vi "Desktop Main.vi"() -> ()   [LabVIEW 2020]
doc: "This template is the Desktop portion of the touch panel template. It is based off of the Queued Message Handler design pattern.\n\nThe Event Handling Loop generates messages based on user interface actions.\n\nThe Message Handling Loop processes messages generated by the Event Handling Loop, or by other messages. The messages are string values, so new messages can be added easily to the Message Cases case structure in the Message Handling Loop. Each message cluster can also provide an optional value for Message Data, which is a variant that can be converted to whatever message-specific data is required.\n\nData is transfered to and from the touch panel target with the use of Shared Variables."
uses:
  controls/UI Data.ctl
  support/Message Queue/Enqueue Message (Single).vi
  <vilib>/Utility/error.llb/Error Cluster From Error Code.vi
  <vilib>/ErrorRing/Error Ring.xnode
  support/Message Queue/Message Queue.lvlib
  support/User Event - Stop/User Event - Stop.lvlib
panel:
  out "Data":dbl(graph)
  in  "Alarm Threshold <Replace Me>":dbl=5.0 format="%#_13g"
  in  "Exit":bool
  # "This template is based off of the Queued Message Handler design pattern.\n\nSee the Queued Message Handler documentation for more information on how to use this design pattern."
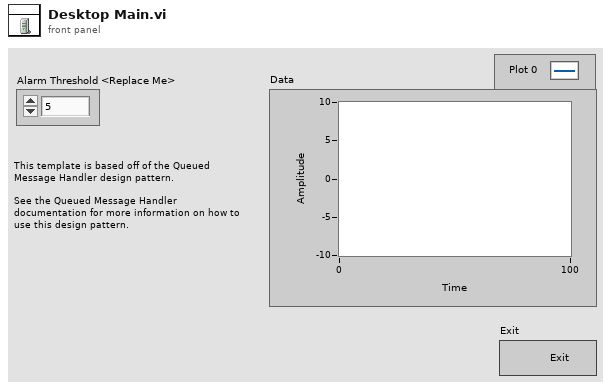
[diagram p1: front panel]
types:
  T1 = typedef "UI Data.ctl" = cluster{"Alarm Threshold <Replace Me>":refnum<vi>, "Exit Button Ref":refnum<vi>}
  T2 = typedef "Message Queue.lvlib/All Message Queues.ctl" = cluster{"UI":refnum<queue>}
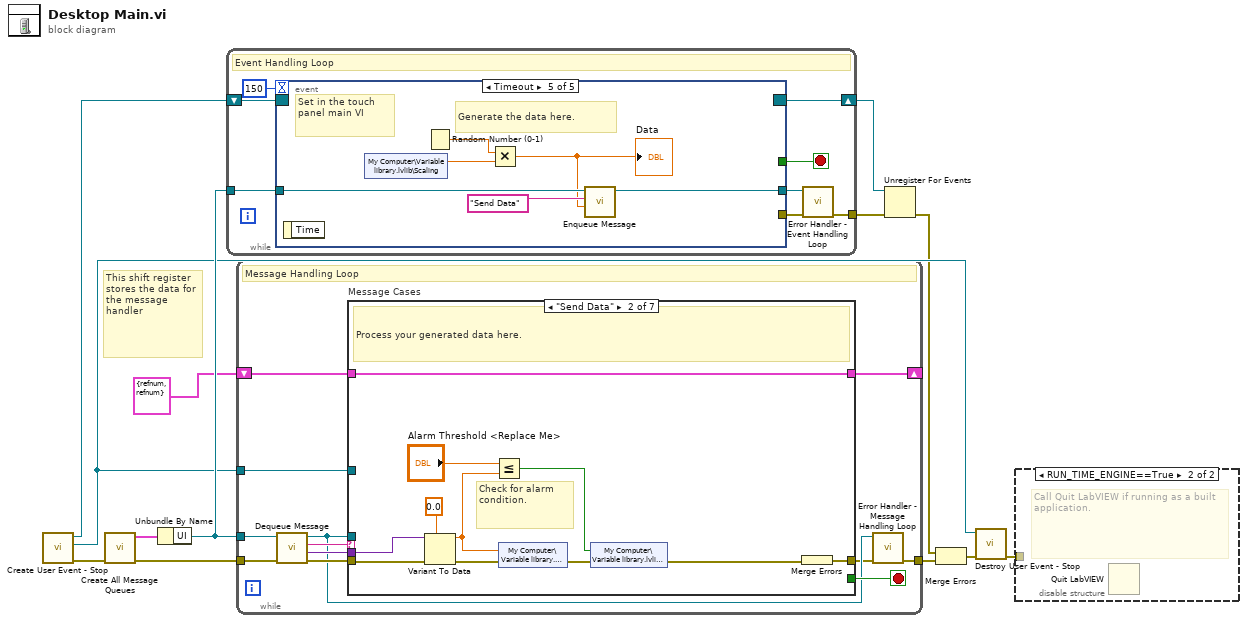
[diagram p0: block diagram]
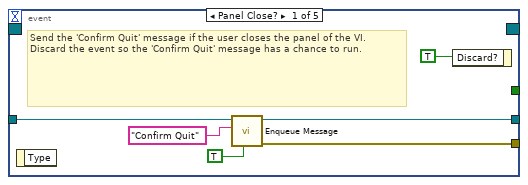
[diagram p3: hidden frame]
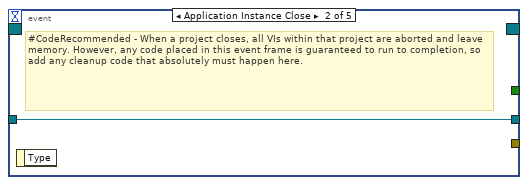
[diagram p4: hidden frame]
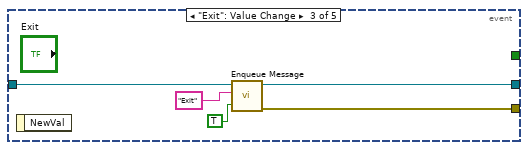
[diagram p5: hidden frame]
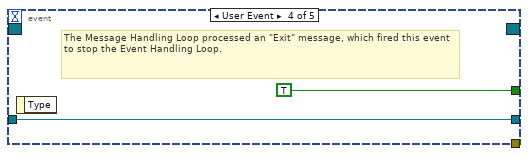
[diagram p6: hidden frame]
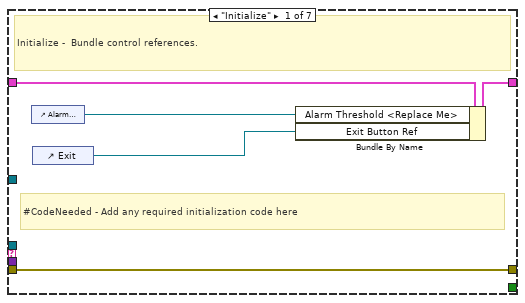
[diagram p7: hidden frame]
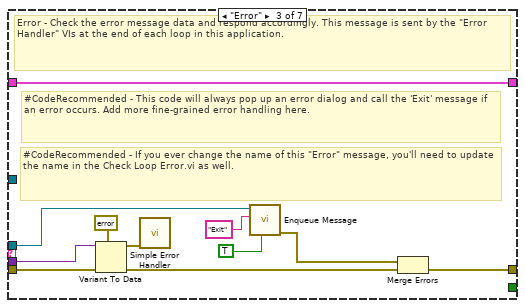
[diagram p8: hidden frame]
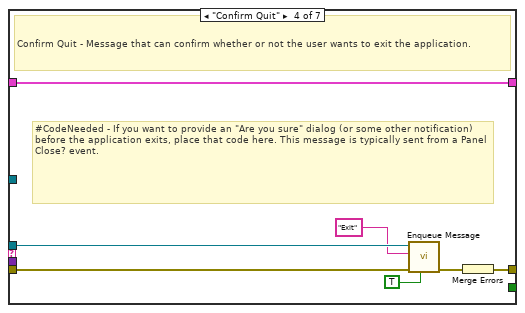
[diagram p9: hidden frame]
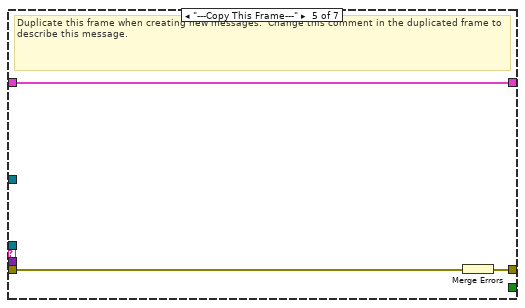
[diagram p10: hidden frame]
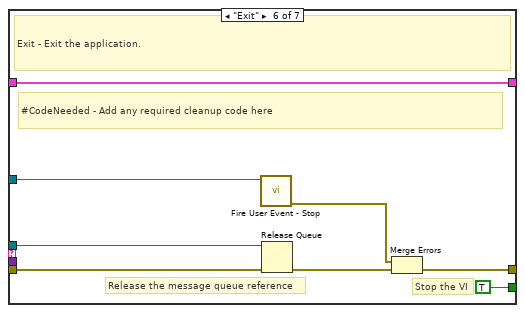
[diagram p11: hidden frame]
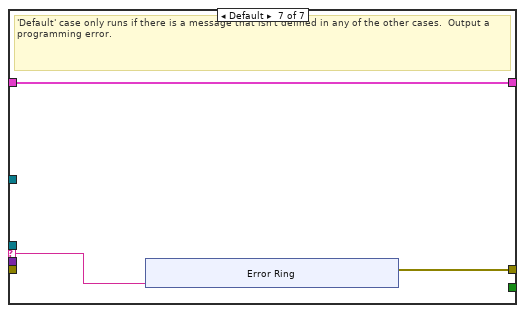
[diagram p12: hidden frame]
diagram:
  # "This shift register stores the data for the message handler"
  n1 = call "Create User Event - Stop.vi"() -> ("error out"=w8:errorcluster, "User Event - Stop"=w6:refnum<user-event>, "Stop Event Registration Refnum"=w9:refnum<event-registration>)  [unwired: 9 in]
  n2 = call "Create All Message Queues.vi"("error in (no error)"=w8) -> ("error out"=w13:errorcluster, "Message Queues out"=w12:T2)  [unwired: 9 in]
  n3 = Unbundle By Name(w12) -> ("UI"=w10:refnum<queue>)
  n4 = while {
    tunnel: w10 -> [w21]
    shift-right: [w19] -> w4
    shift-left: w9 -> [w20]
    tunnel: [w15] -> w1
    stop <- w17 stop-if-true
    # "Event Handling Loop"
    n5 = event shown="[4] Timeout" {
      selector: w20 -> [_ _ _ _ _]
      dyn-events: [_ _ _ _ _] -> w19
      timeout: 150 -> [_ _ _ _ _]
      tunnel: [_ _ _ TRUE ("Discard?") _] -> w17
      tunnel: w21 -> [w26 w28 w33 w35 w41]
      tunnel: [w25 _ w32 _ _] -> w18
      tunnel: [w24 w28 w31 w35 w40] -> w16
      event Panel Close? {
        # "Send the 'Confirm Quit' message if the user closes the panel of the VI. Discard the event so the 'Confirm Quit' message has a chance to run."
        n6 = event-data() -> ()  [unwired: 1 in, 1 out]
        n7 = call-poly "Enqueue Message.vi"("Priority Message? (F)"=TRUE, "Message"="Confirm Quit", "Message Queue"=w26) -> ("error out"=w25:errorcluster, "dup Message Queue"=w24:refnum<queue>)  [unwired: 7 in]
        n8 = event-data("Discard?"=TRUE) -> ()  [unwired: 1 in, 1 out]
      }
      event Application Instance Close {
        # "#CodeRecommended - When a project closes, all VIs within that project are aborted and leave memory. However, any code placed in this event frame is guaranteed to run to completion, so add any cleanup code that absolutely must happen here."
        n9 = event-data() -> ()  [unwired: 1 in, 1 out]
      }
      event "Exit": Value Change {
        n10 = event-data() -> ()  [unwired: 1 in, 1 out]
        n11 = call-poly "Enqueue Message.vi"("Priority Message? (F)"=TRUE, "Message"="Exit", "Message Queue"=w33) -> ("error out"=w32:errorcluster, "dup Message Queue"=w31:refnum<queue>)  [unwired: 7 in]
      }
      event User Event {
        # "The Message Handling Loop processed an \"Exit\" message, which fired this event to stop the Event Handling Loop."
        n12 = event-data() -> ()  [unwired: 1 in, 1 out]
      }
      event Timeout {
        # "Set in the touch panel main VI"
        # "Generate the data here."
        n13 = event-data() -> ()  [unwired: 1 in, 1 out]
        n14 = shared-variable "My Computer\\Variable library.lvlib\\Scaling"() -> (w37:dbl)  [unwired: 1 in, 1 out]
        n15 = Random Number (0-1)() -> (number: 0 to 1=w38:dbl)
        n16 = Multiply(x=w38, y=w37) -> (x*y=w36:dbl)
        "Data" <- w36
        n17 = call-poly "Enqueue Message.vi"("Message Data"=w36, "Message"="Send Data", "Message Queue"=w41) -> ("dup Message Queue"=w40:refnum<queue>)  [unwired: 7 in, 1 out]
      }
    }
    n18 = call "Error Handler - Event Handling Loop.vi"("error in (no error)"=w18, "Message Queue"=w16) -> ("dup error in"=w15:errorcluster)  [unwired: 8 in, 1 out]
  }
  n19 = while {
    tunnel: w10 -> [w45]
    shift-right: [w52] -> _
    shift-left: T1 {"Alarm Threshold <Replace Me>"=refnum, "Exit Button Ref"=refnum} ("Data Cluster") -> [w53]
    tunnel: w6 -> [w50]
    tunnel: w13 -> [w49]
    tunnel: [w43] -> w11
    stop <- w51 stop-if-true
    # "Message Handling Loop"
    n20 = call "Dequeue Message.vi"("error in (no error)"=w49, "Message Queue"=w45) -> ("error out"=w48:errorcluster, "Message Data"=w46:variant, "Message"=w47:string, "dup Message Queue"=w44:refnum<queue>)  [unwired: 6 in]
    n21 = case "Message Cases" shown="\"Send Data\"" w47 {
      selector: w47 -> [_ _ _ _ _ _ w99]
      tunnel: w44 -> [_ _ w72 w83 _ w98 _]
      tunnel: w48 -> [w58 w65 w80 w87 w90 w93 _]
      tunnel: [w58 w68 w73 w85 w88 w94 w100] -> w42
      tunnel: w53 -> [w57 w69 w79 w86 w89 w97 w101]
      tunnel: [w56 w69 w79 w86 w89 w97 w101] -> w52
      tunnel: [_ _ _ _ _ TRUE _] -> w51
      tunnel: w46 -> [_ w63 w78 _ _ _ _]
      tunnel: w50 -> [_ _ _ _ _ w92 _]
      frame "Initialize" {
        # "#CodeNeeded - Add any required initialization code here"
        # "Initialize -  Bundle control references."
        n22 = control-ref of="Alarm Threshold <Replace Me>"() -> (w54:refnum<vi>)
        n23 = control-ref of="Exit"() -> (w55:refnum<vi>)
        n24 = Bundle By Name(cluster=w57, "Alarm Threshold <Replace Me>"=w54, "Exit Button Ref"=w55) -> (w56:T1)
      }
      frame "Send Data" {
        # "Check for alarm condition."
        # "Process your generated data here."
        n25 = Variant To Data(error in=w65, type=0.0 ("Data"), Variant=w63) -> (data=w61:dbl, error out=w60:errorcluster)
        n26 = Less Or Equal?(x="Alarm Threshold <Replace Me>", y=w61) -> (x <= y?=w66:bool)
        n27 = shared-variable "My Computer\\Variable library.lvlib\\Data"(w61, error in=w60) -> (error out=w67:errorcluster)
        n28 = shared-variable "My Computer\\Variable library.lvlib\\Alarm"(w66, error in=w67) -> (error out=w59:errorcluster)
        n29 = Merge Errors(w59) -> (w68:errorcluster)
      }
      frame "Error" {
        # "#CodeRecommended - If you ever change the name of this \"Error\" message, you'll need to update the name in the Check Loop Error.vi as well."
        # "#CodeRecommended - This code will always pop up an error dialog and call the 'Exit' message if an error occurs. Add more fine-grained error handling here."
        # "Error - Check the error message data and respond accordingly. This message is sent by the \"Error Handler\" VIs at the end of each loop in this application."
        n30 = Variant To Data(error in=w80, type=errorcluster {"status"=FALSE, "code"=0, "source"=""} ("error constant"), Variant=w78) -> (data=w76:errorcluster, error out=w75:errorcluster)
        n31 = call <vilib>:"Simple Error Handler.vi"("error in (no error)"=w76) -> ()  [unwired: 4 in, 5 out]
        n32 = call-poly "Enqueue Message.vi"("Priority Message? (F)"=TRUE, "Message"="Exit", "Message Queue"=w72) -> ("error out"=w74:errorcluster)  [unwired: 7 in, 1 out]
        n33 = Merge Errors(w74, w75) -> (w73:errorcluster)
      }
      frame "Confirm Quit" {
        # "#CodeNeeded - If you want to provide an \"Are you sure\" dialog (or some other notification) before the application exits, place that code here. This message is typically sent from a Panel Close? event."
        # "Confirm Quit - Message that can confirm whether or not the user wants to exit the application."
        n34 = call-poly "Enqueue Message.vi"("Priority Message? (F)"=TRUE, "error in (no error)"=w87, "Message"="Exit", "Message Queue"=w83) -> ("error out"=w84:errorcluster)  [unwired: 6 in, 1 out]
        n35 = Merge Errors(w84) -> (w85:errorcluster)
      }
      frame "---Copy This Frame---" {
        # "Duplicate this frame when creating new messages.  Change this comment in the duplicated frame to describe this message."
        n36 = Merge Errors(w90) -> (w88:errorcluster)
      }
      frame "Exit" {
        # "Stop the VI"
        # "Release the message queue reference"
        # "#CodeNeeded - Add any required cleanup code here"
        # "Exit - Exit the application."
        n37 = call "Fire User Event - Stop.vi"("User Event - Stop"=w92) -> ("error out"=w91:errorcluster)  [unwired: 10 in]
        n38 = Release Queue(queue=w98, error in (no error)=w93) -> (error out=w95:errorcluster)  [unwired: 1 in, 2 out]
        n39 = Merge Errors(w91, w95) -> (w94:errorcluster)
      }
      frame Default {
        # "'Default' case only runs if there is a message that isn't defined in any of the other cases.  Output a programming error."
        n40 = xnode "Error Ring"("parameter 0"=w99) -> ("error out"=w100:errorcluster)
      }
    }
    n41 = call "Error Handler - Message Handling Loop.vi"("error in (no error)"=w42, "Message Queue"=w44) -> ("dup error in"=w43:errorcluster)  [unwired: 8 in, 1 out]
  }
  n42 = Unregister For Events(event registration refnum=w4, error in=w1) -> (error out=w5:errorcluster)
  n43 = Merge Errors(w5, w11) -> (w7:errorcluster)
  n44 = call "Destroy User Event - Stop.vi"("error in (no error)"=w7, "User Event - Stop"=w6) -> ("error out"=w2:errorcluster)  [unwired: 9 in]
  n45 = disable-structure shown="RUN_TIME_ENGINE==True" {
    disable-tunnel: w2 -> [_ _]
    frame condition #0 (active) {
    }
    frame condition #1 {
      # "Call Quit LabVIEW if running as a built application."
      n46 = Quit LabVIEW() -> ()  [unwired: 1 in]
    }
  }
